vi "Manage Count.vi"(7 "Inc/Dec":enum16{"Increment", "Decrement"}(ring), 8 "error in (no error)":errorcluster, 10 "Relay Indexes":i32[](array[numeric]), 11 "SLSC Switch in":refnum<class "SLSC Switch.lvclass">) -> (0 "error out":errorcluster, 1 "Relay Counts":i32[](array[numeric]), 3 "SLSC Switch out":refnum<class "SLSC Switch.lvclass">)   [LabVIEW 2016, in "SLSC Switch.lvlib" / "SLSC Switch.lvclass"]
uses:
  SLSC Switch.lvclass
  SLSC Switch.lvclass/SLSC Switch.ctl
  Switch Action Processor/Switch Action Processor.lvclass
  Relay/Relay.lvclass
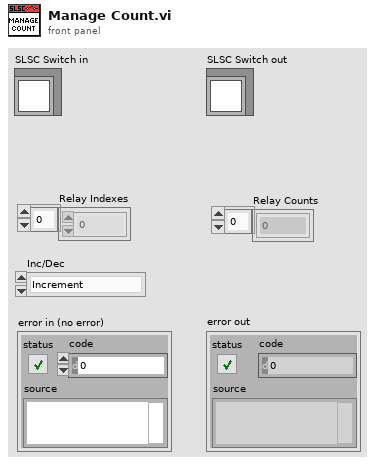
[diagram p1: front panel]
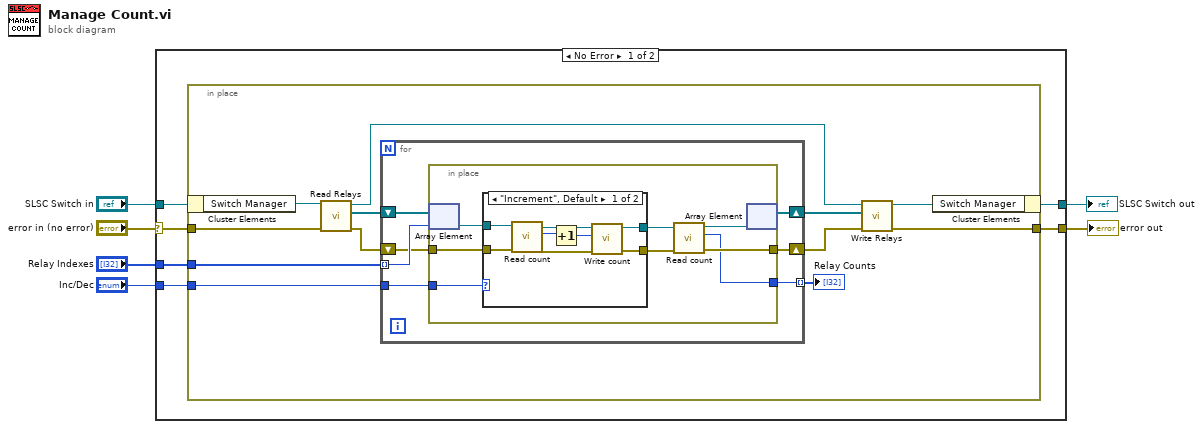
[diagram p0: block diagram]
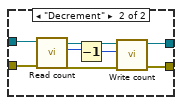
[diagram p2: hidden frame]
diagram:
  n1 = case shown="No Error" "error in (no error)" {
    selector: "error in (no error)" -> [w10 w57]
    tunnel: "Relay Indexes" -> [w12 _]
    tunnel: [w11 w57] -> w5
    tunnel: "SLSC Switch in" -> [w9 w56]
    tunnel: [w8 w56] -> w2
    tunnel: "Inc/Dec" -> [w7 _]
    frame No Error {
      n2 = in-place {
        in-place-border: w12 -> [w22]
        in-place-border: [w21] -> w11
        in-place-border: w10 -> [w16]
        in-place-border: w7 -> [w13]
        n3 = in-place-cluster #1(w9) -> ("Switch Manager"=w15:refnum<class "Switch Action Processor.lvclass">)
        n4 = call-dynamic "Read Relays.vi"("error in (no error)"=w16, "Switch Action Processor in"=w15) -> ("error out"=w17:errorcluster, "Relays"=w18:refnum<class "Relay.lvclass">[], "Switch Action Processor out"=w19:refnum<class "Switch Action Processor.lvclass">)  [unwired: 7 in]
        n5 = for {
          tunnel: w22 -> [w30] mode=indexing
          shift-right: [w27] -> w24
          shift-left: w18 -> [w31]
          shift-right: [w28] -> w23
          shift-left: w17 -> [w29]
          tunnel: [w26] -> w20 mode=indexing
          tunnel: w13 -> [w25]
          n6 = in-place {
            in-place-border: w29 -> [w38]
            in-place-border: [w34] -> w28
            in-place-border: [w33] -> w26
            in-place-border: w25 -> [w32]
            n7 = in-place-array #2(w31, w30) -> (w39:refnum<class "Relay.lvclass">)
            n8 = case shown="\"Increment\", Default" w32 {
              tunnel: w39 -> [w43 w51]
              tunnel: [w42 w48] -> w37
              tunnel: w38 -> [w41 w50]
              tunnel: [w40 w49] -> w36
              frame "Increment", Default {
                n9 = call-dynamic "Read count.vi"("error in (no error)"=w41, "Relay in"=w43) -> ("error out"=w46:errorcluster, "count"=w47:i32, "Relay out"=w45:refnum<class "Relay.lvclass">)  [unwired: 7 in]
                n10 = Increment(x=w47) -> (x+1=w44:i32)
                n11 = call-dynamic "Write count.vi"("error in (no error)"=w46, "count"=w44, "Relay in"=w45) -> ("error out"=w40:errorcluster, "Relay out"=w42:refnum<class "Relay.lvclass">)  [unwired: 7 in]
              }
              frame "Decrement" {
                n12 = call-dynamic "Read count.vi"("error in (no error)"=w50, "Relay in"=w51) -> ("error out"=w54:errorcluster, "count"=w55:i32, "Relay out"=w53:refnum<class "Relay.lvclass">)  [unwired: 7 in]
                n13 = Decrement(x=w55) -> (x-1=w52:i32)
                n14 = call-dynamic "Write count.vi"("error in (no error)"=w54, "count"=w52, "Relay in"=w53) -> ("error out"=w49:errorcluster, "Relay out"=w48:refnum<class "Relay.lvclass">)  [unwired: 7 in]
              }
            }
            n15 = call-dynamic "Read count.vi"("error in (no error)"=w36, "Relay in"=w37) -> ("error out"=w34:errorcluster, "count"=w33:i32, "Relay out"=w35:refnum<class "Relay.lvclass">)  [unwired: 7 in]
            n16 = in-place-array #2(w35) -> (w27:refnum<class "Relay.lvclass">[])  [unwired: 1 out]
          }
        }
        "Relay Counts" <- w20
        n17 = call-dynamic "Write Relays.vi"("error in (no error)"=w23, "Relays"=w24, "Switch Action Processor in"=w19) -> ("error out"=w21:errorcluster, "Switch Action Processor out"=w14:refnum<class "Switch Action Processor.lvclass">)  [unwired: 7 in]
        n18 = in-place-cluster #1("Switch Manager"=w14) -> (w8:refnum<class "SLSC Switch.lvclass">)
      }
    }
    frame Error {
    }
  }
  "error out" <- w5
  "SLSC Switch out" <- w2
